vi "appendRun.vi"(4 "Style":refnum<class "Style.lvclass">, 6 "value":string, 8 "error in (no error)":errorcluster, 11 "Paragraph in":refnum<k24>) -> (0 "error out":errorcluster, 3 "reference out":refnum<k24>)   [LabVIEW 2017, in "xwpfWriter.lvclass"]
uses:
  xwpfWriter.lvclass
  C:/Users/Neo/Desktop/Dev_Tools_BR/LabVIEW_NPOI/src/lib/NPOI 2.1.1/NPOI.OOXML.dll
  lib/NPOI 2.1.1/NPOI.OOXML.dll
  Styles/Style/Style.lvclass
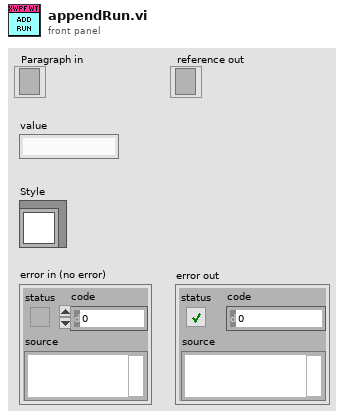
[diagram p1: front panel]
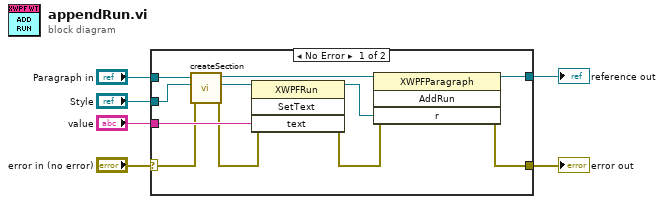
[diagram p0: block diagram]
diagram:
  n1 = case shown="No Error" "error in (no error)" {
    selector: "error in (no error)" -> [w9 w19]
    tunnel: "value" -> [w14 _]
    tunnel: "Paragraph in" -> [w13 w18]
    tunnel: "Style" -> [w12 _]
    tunnel: [w8 w18] -> w2
    tunnel: [w7 w19] -> w1
    frame No Error {
      n2 = call "createSection.vi"("error in (no error)"=w9, "Style"=w12, "Paragraph in"=w13) -> ("error out"=w11:errorcluster, "Section out"=w16:refnum<k24>, "Paragraph out"=w17:refnum<k24>)  [unwired: 6 in]
      n3 = invoke class="XWPFRun" method="SetText"(reference=w16, error in=w11, "text"=w14) -> (reference out=w15:refnum<k24>, error out=w10:errorcluster)  [unwired: 1 in, 2 out]
      n4 = invoke class="XWPFParagraph" method="AddRun"(reference=w17, error in=w10, "r"=w15) -> (reference out=w8:refnum<k24>, error out=w7:errorcluster)  [unwired: 1 in, 2 out]
    }
    frame Error {
    }
  }
  "reference out" <- w2
  "error out" <- w1
